vi "Get AI REF (f) StringsAndValues.vi"(8 "error in (no error)":errorcluster, 10 "Channels.REF":T1 {"Roll-Off" min=1; "TC" min=0.0001 format="%#_3p"; "Phase" format="%#_3g"; "Frequency" min=0.0001 max=200000.0 format="%#_6p"; "Channel" min=1}, 11 "Configuration.DAQ":T3 {"AO terminal config" items=[""=-1, "differential"=10106, "pseudodifferential"=12529]; "AI terminal config" items=[""=-1, "differential"=10106, "pseudodifferential"=12529]; "AI.Coupling" items=[""=0, "AC"=10045, "DC"=10050, "GND"=10066]}) -> (0 "error out":errorcluster, 2 "AI REF (f) StringsAndValues":cluster{string, i32}[](array[cluster]))   [LabVIEW 2019, in "Instrument.Lockin.lvlib" / "Instrument UI.Lockin.lvclass"]
uses:
  Instrument UI.Lockin.lvclass
  Instrument.DAQ/Typedefs/DAQ.Configuration--Cluster--Array.ctl
  Instrument.DAQ/Typedefs/DAQ.Configuration--Cluster.ctl
  Instrument.DAQ/Typedefs/DAQ.Config.AO.Range--enum.ctl
  Instrument.DAQ/Typedefs/DAQ.Config.AI.Range--enum.ctl
  Instrument.DAQ/Typedefs/DAQ.Config.AI.Coupling--enum.ctl
  Instrument.DAQ/Typedefs/DAQ.TerminalConfiguration--ring.ctl
  Instrument.DAQ/Typedefs/REF.Channel--Cluster--Array.ctl
  Instrument.DAQ/Typedefs/REF.Channel--Cluster.ctl
  Instrument.DAQ/Instrument.DAQ.lvclass
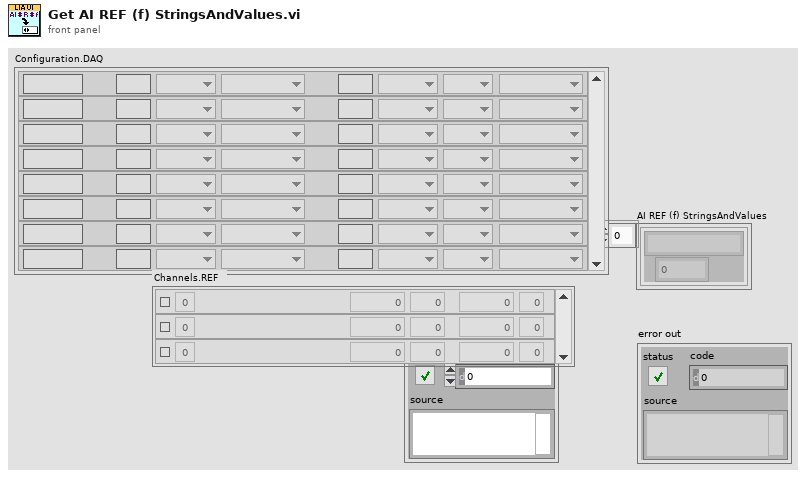
[diagram p1: front panel]
types:
  T1 = typedef "Instrument.Lockin.lvlib/Instrument.DAQ.lvclass/REF.Channel--Cluster--Array.ctl" = T2[]
  T2 = typedef "Instrument.Lockin.lvlib/Instrument.DAQ.lvclass/REF.Channel--Cluster.ctl" = cluster{"Enable?":bool, "Channel":i32, "Frequency":dbl, "Phase":dbl, "TC":dbl, "Roll-Off":i32}
  T3 = typedef "Instrument.Lockin.lvlib/Instrument.DAQ.lvclass/DAQ.Configuration--Cluster--Array.ctl" = T4[]
  T4 = typedef "Instrument.Lockin.lvlib/Instrument.DAQ.lvclass/DAQ.Configuration--Cluster.ctl" = cluster{"Device":string, "AO.Ch":string, "AO.Range":T5, "AI.Ch":string, "AI.Range":T6, "AI.Coupling":T7, "AI terminal config":T8, "AO terminal config":T8}
  T5 = typedef "Instrument.Lockin.lvlib/Instrument.DAQ.lvclass/DAQ.Config.AO.Range--enum.ctl" = enum16{"±0.1", "±1.0", "±10.0", ""}
  T6 = typedef "Instrument.Lockin.lvlib/Instrument.DAQ.lvclass/DAQ.Config.AI.Range--enum.ctl" = enum16{"±0.316", "±1.00", "±3.16", "±10.0", "±31.6", "±42.4", ""}
  T7 = typedef "Instrument.Lockin.lvlib/Instrument.DAQ.lvclass/DAQ.Config.AI.Coupling--enum.ctl" = u16
  T8 = typedef "Instrument.Lockin.lvlib/Instrument.DAQ.lvclass/DAQ.TerminalConfiguration--ring.ctl" = i32
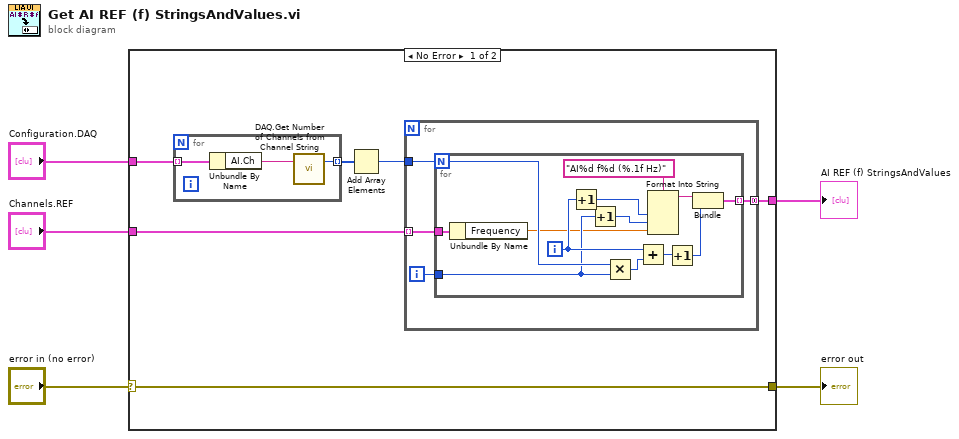
[diagram p0: block diagram]
diagram:
  n1 = case shown="No Error" "error in (no error)" {
    selector: "error in (no error)" -> [w9 w32]
    tunnel: [w10 _] -> w5
    tunnel: [w9 w32] -> w3
    tunnel: "Channels.REF" -> [w7 _]
    tunnel: "Configuration.DAQ" -> [w6 _]
    frame No Error {
      n2 = for {
        tunnel: w6 -> [w14] mode=indexing
        tunnel: [w13] -> w11 mode=indexing
        n3 = Unbundle By Name(w14) -> ("AI.Ch"=w12:string)
        n4 = call "DAQ.Get Number of Channels from Channel String.vi"("Channels String"=w12) -> ("# channels"=w13:i32)  [unwired: 2 in]
      }
      n5 = Add Array Elements(numeric array=w11) -> (sum=w8:i32)
      n6 = for {
        tunnel: w7 -> [w16] mode=indexing
        tunnel: [w17] -> w10 mode=concatenating
        tunnel: w8 -> [w15]
        i -> [w18]
        n7 = for {
          N: w15 -> [w26]
          tunnel: [w31] -> w17 mode=indexing
          tunnel: w18 -> [w23]
          tunnel: w16 -> [w21]
          i -> [w24]
          n8 = Unbundle By Name(w21) -> ("Frequency"=w20:dbl)
          n9 = Increment(x=w24) -> (x+1=w19:i32)
          n10 = Increment(x=w23) -> (x+1=w22:i32)
          n11 = Multiply(x=w26, y=w23) -> (x*y=w25:i32)
          n12 = Add(x=w24, y=w25) -> (x+y=w30:i32)
          n13 = Format Into String(format string="AI%d f%d (%.1f Hz)", w19, w22, w20) -> (resulting string=w28:string)  [unwired: 2 in, 1 out]
          n14 = Increment(x=w30) -> (x+1=w27:i32)
          n15 = Bundle(w28, w27) -> (w31:cluster{string, i32})  [unwired: 1 in]
        }
      }
    }
    frame Error {
    }
  }
  "AI REF (f) StringsAndValues" <- w5
  "error out" <- w3
